vi "RF with WF Sweep.vi"() -> ()   [LabVIEW 2012]
uses:
  <vilib>/DAQmx/read.llb/DAQmx Read (Counter U32 1Chan 1Samp).vi
  <vilib>/Utility/file.llb/Write To Spreadsheet File (DBL).vi
  <vilib>/DAQmx/miscellaneous.llb/DAQmx Fill In Error Info.vi
  <vilib>/DAQmx/create/channels.llb/DAQmx Create Channel (CI-Count Edges).vi
  <vilib>/DAQmx/create/channels.llb/DAQmx Create Channel (CO-Pulse Generation-Ticks).vi
  <vilib>/DAQmx/configure/timing.llb/DAQmx Timing (Implicit).vi
  <vilib>/DAQmx/configure/timing.llb/DAQmx Timing (Sample Clock).vi
  <resource>/objmgr/daqmx.rc
panel:
  out "Scan":i32=222
  in  "N Scans":i32=100
  out "freq":dbl=349000000.0
  out "diff":dbl=487.0
  out "loop":i32=99
  in  "file path (dialog if empty)":path
  out "Z Position 2":dbl=39.24
  out "Y Position 2":dbl=141.00216667506004
  out "X Position 2":dbl=-28.668339852561274
  in  "CW for tracking":bool
  in  "Y Parameters":T1={"Number of Y Steps"=200, "Max Y (V)"=2.0, "Min Y (V)"=-2.0}
  in  "X":T2={"Number of X Steps"=200, "Max X (V)"=2.0, "Min X (V)"=-2.0}
  in  "Z Position":dbl=39.24
  in  "Y Position":dbl=136.0
  in  "X Position":dbl=-24.0
  in  "Z-track?":bool=TRUE
  out "XY Graph":cluster{"Y":dbl[], "Y":dbl[]}[](graph)=[{"Y"=[250000000.0, 251000000.0, 252000000.0, 253000000.0, 254000000.0, 255000000.0, 256000000.0, 257000000.0, 258000000.0, 259000000.0, 260000000.0, 261000000.0, 262000000.0, 263000000.0, 264000000.0, 265000000.0, 266000000.0, 267000000.0, 268000000.0, 269000000.0, 270000000.0, 271000000.0, 272000000.0, 273000000.0, 274000000.0, 275000000.0, 276000000.0, 277000000.0, 278000000.0, 279000000.0, 280000000.0, 281000000.0, 282000000.0, 283000000.0, 284000000.0, 285000000.0, 286000000.0, 287000000.0, 288000000.0, 289000000.0, 290000000.0, 291000000.0, 292000000.0, 293000000.0, 294000000.0, 295000000.0, 296000000.0, 297000000.0, 298000000.0, 299000000.0, 300000000.0, 301000000.0, 302000000.0, 303000000.0, 304000000.0, 305000000.0, 306000000.0, 307000000.0, 308000000.0, 309000000.0, 310000000.0, 311000000.0, 312000000.0, 313000000.0, 314000000.0, 315000000.0, 316000000.0, 317000000.0, 318000000.0, 319000000.0, 320000000.0, 321000000.0, 322000000.0, 323000000.0, 324000000.0, 325000000.0, 326000000.0, 327000000.0, 328000000.0, 329000000.0, 330000000.0, 331000000.0, 332000000.0, 333000000.0, 334000000.0, 335000000.0, 336000000.0, 337000000.0, 338000000.0, 339000000.0, 340000000.0, 341000000.0, 342000000.0, 343000000.0, 344000000.0, 345000000.0, 346000000.0, 347000000.0, 348000000.0, 349000000.0], "Y"=[109367.0, 118171.0, 118039.0, 118323.0, 118900.0, 117820.0, 117949.0, 118621.0, 118408.0, 118705.0, 117982.0, 118762.0, 119039.0, 119174.0, 119042.0, 119150.0, 118801.0, 118275.0, 118226.0, 119115.0, 118390.0, 118344.0, 118771.0, 118925.0, 118432.0, 118761.0, 118837.0, 118494.0, 117973.0, 117930.0, 118009.0, 118829.0, 118281.0, 119222.0, 118046.0, 117569.0, 117633.0, 117115.0, 116624.0, 116136.0, 115617.0, 116138.0, 116137.0, 116297.0, 115963.0, 116921.0, 117750.0, 117966.0, 118454.0, 117806.0, 117382.0, 116437.0, 117111.0, 116829.0, 116627.0, 115825.0, 116660.0, 116366.0, 116608.0, 116374.0, 116876.0, 116660.0, 117066.0, 116940.0, 116833.0, 117718.0, 117672.0, 118037.0, 118493.0, 118553.0, 118497.0, 117416.0, 118662.0, 117772.0, 118756.0, 117519.0, 117715.0, 118588.0, 117434.0, 117658.0, 117836.0, 118066.0, 118672.0, 118019.0, 118259.0, 118223.0, 118716.0, 118339.0, 117569.0, 118481.0, 118298.0, 118509.0, 118430.0, 117846.0, 117520.0, 117628.0, 118067.0, 118519.0, 118455.0, 117629.0]}]
  in  "Freq Max":dbl=350000000.0
  in  "Freq  Step":dbl=1000000.0
  in  "Freq Min":dbl=250000000.0
  in  "power":dbl=-9.0
  in  "stop":bool
  in  "Path to spinapi.dll":path=path "C:/SpinCore/SpinAPI/dll/spinapi64.dll"
  in  "Pulse offset":dbl
  in  "Tau":dbl=5e-07
  in  "RF Pulse":dbl=1e-07
  in  "Rabi Freq":dbl=11750000.0
  in  "MW Delay":dbl=2e-08
  in  "APD signal width":dbl=3e-07
  in  "Signal Delay":dbl=7.6e-07
  in  "AOM Rest time":dbl=1e-06
  in  "AOM Pulse length":dbl=2.5e-06
  in  "N Loop":i32=100000
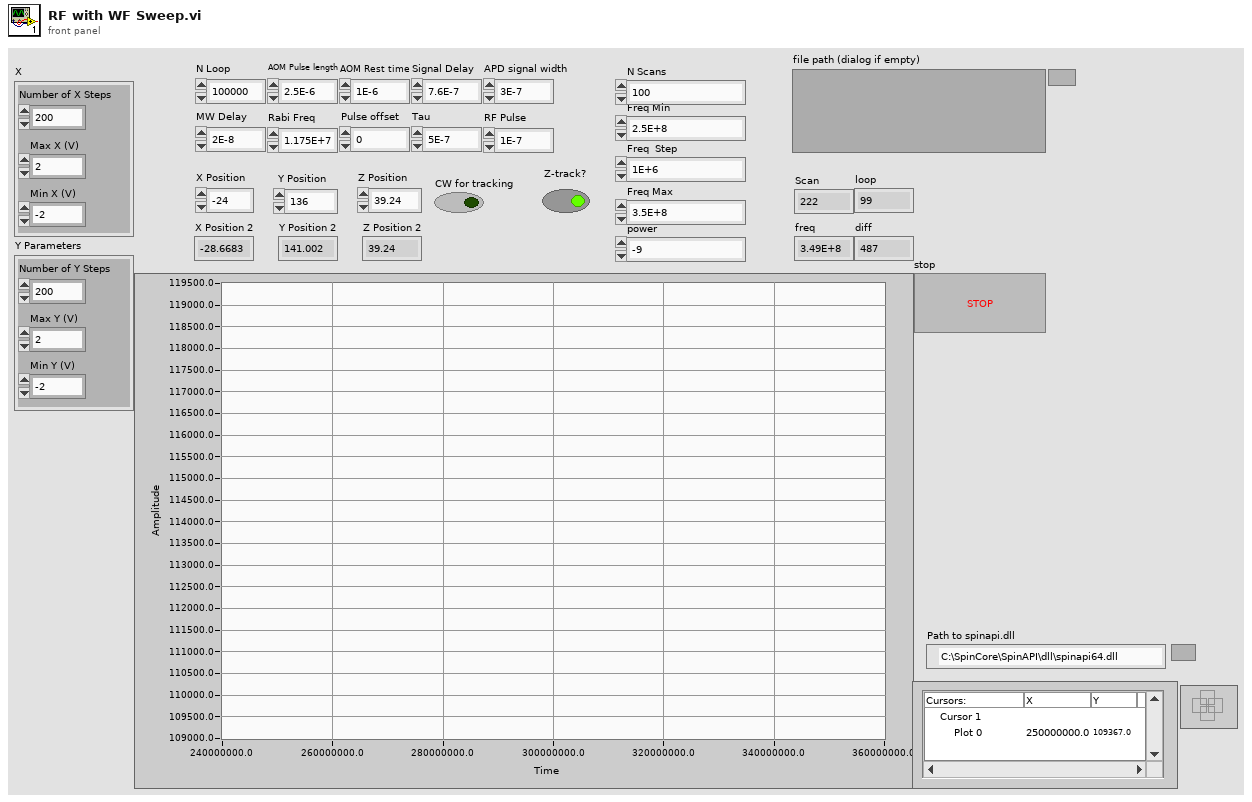
[diagram p1: front panel]
types:
  T1 = cluster{"Number of Y Steps":i32, "Max Y (V)":dbl, "Min Y (V)":dbl}
  T2 = cluster{"Number of X Steps":i32, "Max X (V)":dbl, "Min X (V)":dbl}
  T3 = enum16{"Pulse Program", "Frequency Registers", "TX Phase Registers", "RX Phase Registers"}
  T4 = cluster{"Instruct Data":i32, "Op Code":i32, "Flags":bool[], "Comments":string, "Time (s)":dbl}[]
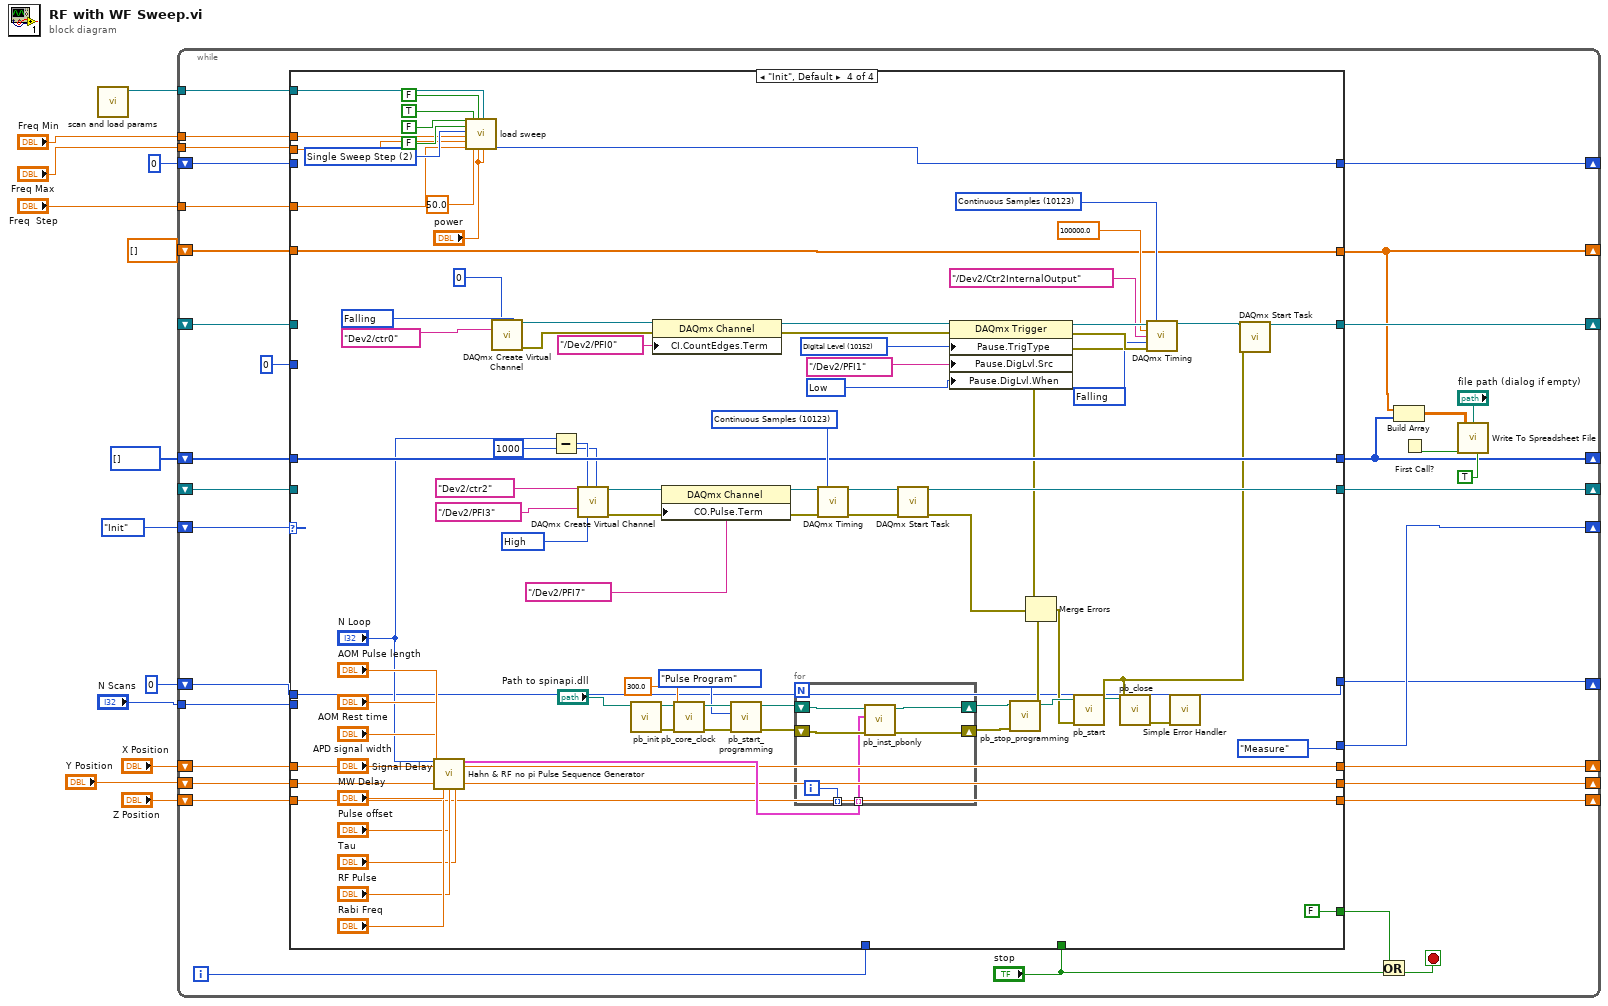
[diagram p0: block diagram]
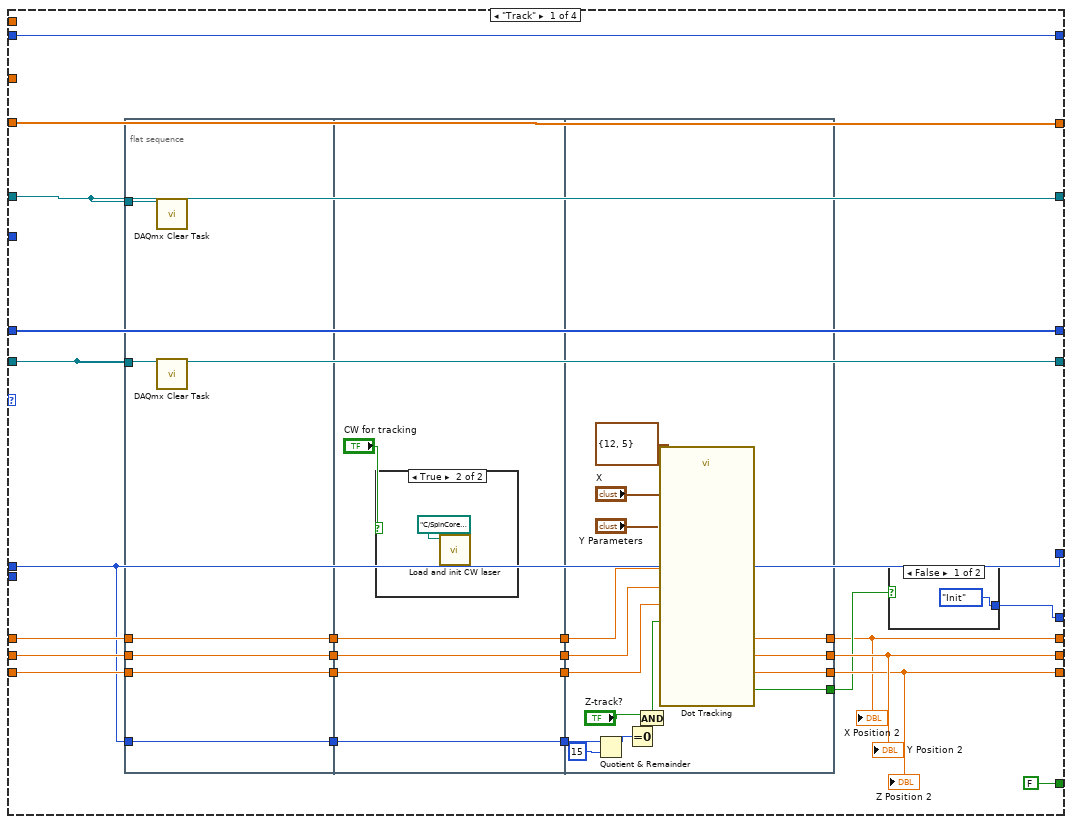
[diagram p2: hidden frame]
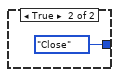
[diagram p3: hidden frame]
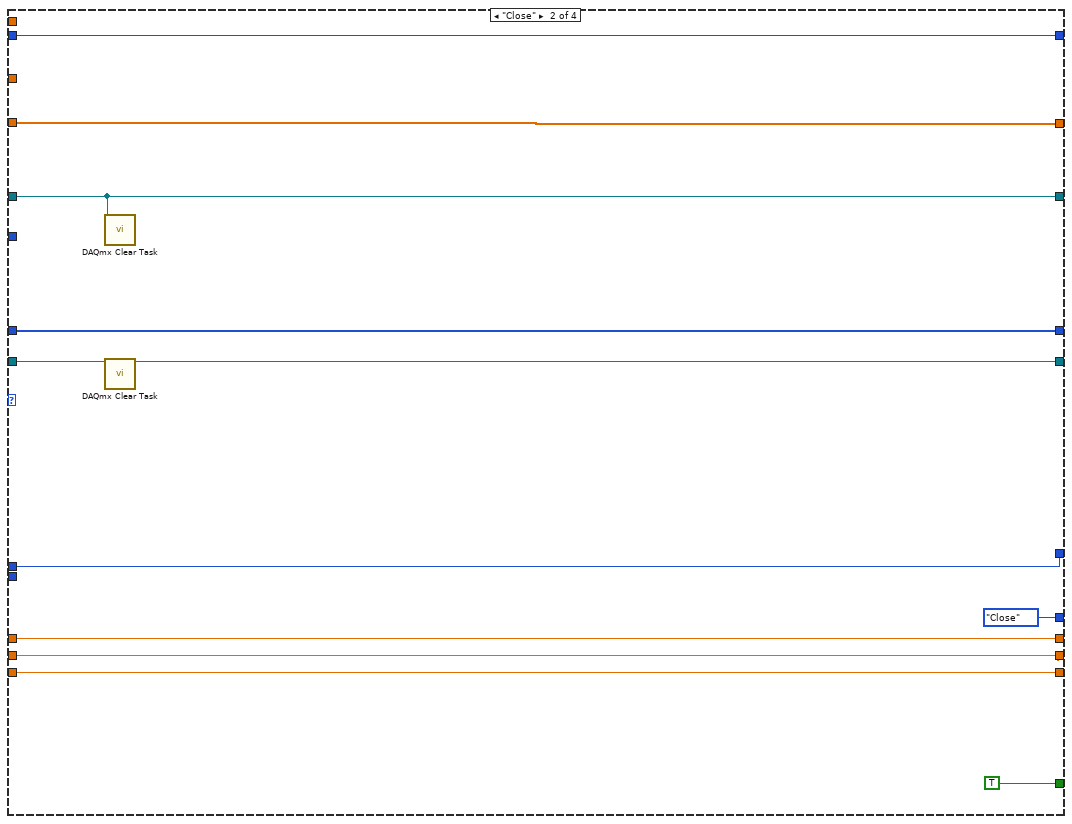
[diagram p5: hidden frame]
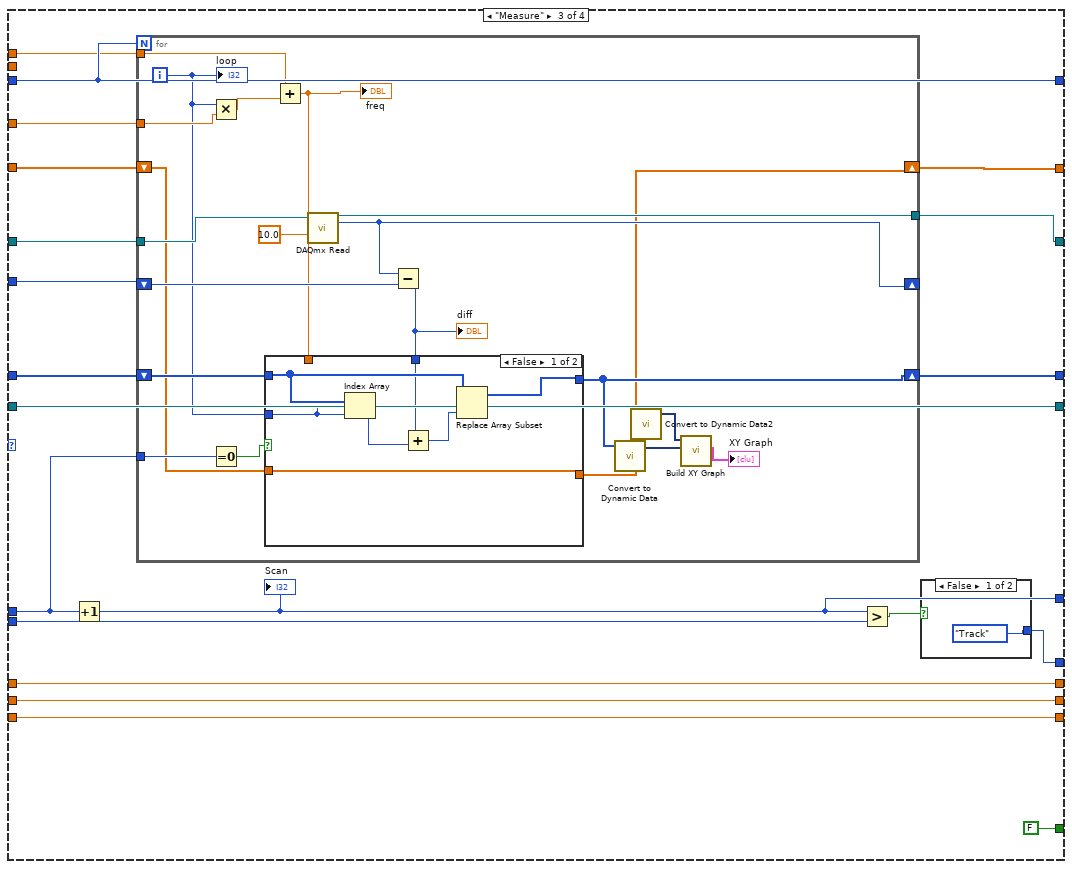
[diagram p6: hidden frame]
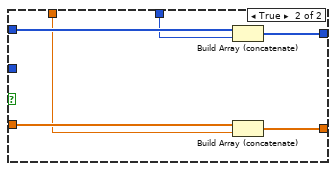
[diagram p7: hidden frame]
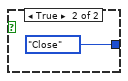
[diagram p8: hidden frame]
diagram:
  n1 = call "scan and load params.vi"() -> ("Serial Port Select"=w7:refnum<visa-resource-name>)  [unwired: 9 out]
  n2 = while {
    shift-right: [w41] -> _
    shift-left: enum16{"Init", "Track", "Measure", "Close", ""}."Init" -> [w47]
    shift-right: [w46] -> _
    shift-left: _ -> [w34]
    shift-right: [w45] -> _
    shift-left: _ -> [w35]
    shift-right: [w16] -> _
    shift-left: u32[] [] -> [w43]
    shift-right: [w29] -> _
    shift-left: dbl[] [] -> [w42]
    shift-right: [w40] -> _
    shift-left: "X Position" -> [w31]
    shift-right: [w39] -> _
    shift-left: "Y Position" -> [w37]
    shift-right: [w38] -> _
    shift-left: "Z Position" -> [w36]
    tunnel: w7 -> [w24]
    tunnel: "Freq  Step" -> [w21]
    tunnel: "Freq Max" -> [w22]
    tunnel: "Freq Min" -> [w23]
    shift-right: [w20] -> _
    shift-left: u16 0 ("Number\nof Points") -> [w19]
    tunnel: "N Scans" -> [w18]
    shift-right: [w15] -> _
    shift-left: 0 -> [w17]
    i -> [w14]
    stop <- w33 stop-if-true
    n3 = case shown="\"Init\", Default" w47 {
      tunnel: [w54 w111 w125 w196] -> w46
      tunnel: [w53 w110 w118 w195] -> w45
      tunnel: "stop" -> [_ _ _ _]
      tunnel: w43 -> [w63 w109 w131 w193]
      tunnel: w42 -> [w58 w104 w130 w189]
      tunnel: [w63 w109 w129 w193] -> w16
      tunnel: [w58 w104 w122 w189] -> w29
      tunnel: [w62 enum16{"Init", "Track", "Measure", "Close", ""}."Close" w128 enum16{"Init", "Track", "Measure", "Close", ""}."Measure"] -> w41
      tunnel: [w51 w103 w121 w188] -> w40
      tunnel: [w70 w108 w124 w191] -> w39
      tunnel: [w69 w107 w123 w190] -> w38
      tunnel: w37 -> [w66 w108 w124 w191]
      tunnel: w36 -> [w64 w107 w123 w190]
      tunnel: w35 -> [w53 w110 w126 _]
      tunnel: w34 -> [w54 w111 w125 _]
      tunnel: [FALSE TRUE FALSE FALSE] -> w32
      tunnel: w31 -> [w59 w103 w121 w188]
      tunnel: u32 0 ("data") -> [_ _ w120 _]
      tunnel: w24 -> [_ _ _ w181]
      tunnel: w23 -> [_ _ w117 w173]
      tunnel: w22 -> [_ _ _ w172]
      tunnel: w21 -> [_ _ w116 w171]
      tunnel: [w52 w102 w119 w170] -> w20
      tunnel: w19 -> [w52 w102 w119 _]
      tunnel: w18 -> [_ _ w114 _]
      tunnel: w17 -> [w50 w101 w112 w169]
      tunnel: [w50 w101 w113 w169] -> w15
      tunnel: w14 -> [_ _ _ _]
      frame "Track" {
        n4 = flat-sequence {
          tunnel: w64 -> [w76]
          tunnel: w66 -> [w77]
          tunnel: w59 -> [w78]
          tunnel: [w78] -> w57
          tunnel: [w77] -> w56
          tunnel: [w76] -> w55
          tunnel: w54 -> [w75]
          tunnel: w53 -> [w74]
          tunnel: w50 -> [w73]
          tunnel: [w73] -> w49
          tunnel: [w83] -> w68
          tunnel: [w82] -> w67
          tunnel: [w81] -> w65
          tunnel: w57 -> [w83]
          tunnel: w56 -> [w82]
          tunnel: w55 -> [w81]
          tunnel: w49 -> [w79]
          tunnel: [w79] -> w48
          tunnel: [w100] -> w51
          tunnel: [w99] -> w70
          tunnel: [w98] -> w69
          tunnel: w68 -> [w97]
          tunnel: w67 -> [w96]
          tunnel: w65 -> [w95]
          tunnel: [w91] -> w61
          tunnel: w48 -> [w85]
          frame #0 {
            n5 = call <vilib>:"DAQmx Clear Task.vi"("task in"=w74) -> ()  [unwired: 14 in, 1 out]
            n6 = call <vilib>:"DAQmx Clear Task.vi"("task in"=w75) -> ()  [unwired: 14 in, 1 out]
          }
          frame #1 {
            n7 = case shown="True" "CW for tracking" {
              frame False {
              }
              frame True {
                n8 = call "Load and init CW laser.vi"("path in"=path "C:/SpinCore/SpinAPI/dll/spinapi64.dll") -> ()  [unwired: 11 in]
              }
            }
          }
          frame #2 {
            n9 = Quotient & Remainder(x=w85, y=15) -> (x-y*floor(x/y)=w89:i32)  [unwired: 1 out]
            n10 = Equal To 0?(x=w89) -> (x = 0?=w88:bool)
            n11 = And(x="Z-track?", y=w88) -> (x .and. y?=w86:bool)
            n12 = call "Dot Tracking.vi"("X"="X", "Y Parameters"="Y Parameters", "RS232 settings"=cluster{"Portnumber":i32, "Baudrate":u16} {"Portnumber"=12, "Baudrate"=5}, "X Pos"=w97, "Y pos"=w96, "Z Pos"=w95, "Z-track?"=w86) -> ("X Position"=w100:dbl, "Y Position"=w99:dbl, "Z Position"=w98:dbl, "Gave up?"=w91:bool)  [unwired: 2 in, 3 out]
          }
        }
        n13 = case shown="False" w61 {
          tunnel: [enum16{"Init", "Track", "Measure", "Close", ""}."Init" enum16{"Init", "Track", "Measure", "Close", ""}."Close"] -> w62
          frame False {
          }
          frame True {
          }
        }
        "X Position 2" <- w51
        "Y Position 2" <- w70
        "Z Position 2" <- w69
      }
      frame "Close" {
        n14 = call <vilib>:"DAQmx Clear Task.vi"("task in"=w110) -> ()  [unwired: 14 in, 1 out]
        n15 = call <vilib>:"DAQmx Clear Task.vi"("task in"=w111) -> ()  [unwired: 14 in, 1 out]
      }
      frame "Measure" {
        n16 = Increment(x=w112) -> (x+1=w113:i32)
        "Scan" <- w113
        n17 = for {
          N: w119 -> [_]
          shift-right: [w142] -> w129
          shift-left: w131 -> [w143]
          shift-right: [w133] -> w122
          shift-left: w130 -> [w134]
          tunnel: w126 -> [w150]
          shift-right: [w145] -> _
          shift-left: w120 -> [w147]
          tunnel: [w146] -> w118
          tunnel: w117 -> [w141]
          tunnel: w116 -> [w140]
          tunnel: w112 -> [w137]
          i -> [w135]
          n18 = Multiply(x=w135, y=w140) -> (x*y=w139:dbl)
          n19 = Equal To 0?(x=w137) -> (x = 0?=w136:bool)
          n20 = Add(x=w141, y=w139) -> (x+y=w132:dbl)
          "freq" <- w132
          n21 = call-poly <vilib>:"DAQmx Read.vi"("task/channels in"=w150, "timeout"=10.0) -> ("task out"=w146:refnum<k21>, "data"=w145:u32)  [unwired: 11 in, 1 out]
          n22 = Subtract(x=w145, y=w147) -> (x-y=w138:u32)
          "diff" <- w138
          n23 = case shown="False" w136 {
            tunnel: w143 -> [w158 w164]
            tunnel: [w153 w163] -> w142
            tunnel: w138 -> [w155 w162]
            tunnel: w135 -> [w157 _]
            tunnel: w134 -> [w152 w161]
            tunnel: [w152 w160] -> w133
            tunnel: w132 -> [_ w159]
            frame False {
              n24 = Index Array(array=w158, index=w157) -> (element=w156:u32)
              n25 = Add(x=w155, y=w156) -> (x+y=w154:u32)
              n26 = Replace Array Subset(array=w158, new element=w154, index=w157) -> (w153:u32[])
            }
            frame True {
              n27 = Build Array (concatenate)(w164, w162) -> (w163:u32[])
              n28 = Build Array (concatenate)(w161, w159) -> (w160:dbl[])
            }
          }
          n29 = call "Convert to Dynamic Data"("Array"=w142) -> ("Dynamic Data Type"=w148:dynamicdata)  [unwired: 3 in]
          n30 = call "Convert to Dynamic Data2"("Array"=w133) -> ("Dynamic Data Type"=w149:dynamicdata)  [unwired: 3 in]
          n31 = call "Build XY Graph"("Y Input"=w148, "X Input"=w149) -> ("XY Graph"=→"XY Graph":cluster{"Y":dbl[], "Y":dbl[]}[])  [unwired: 3 in, 6 out]
          "loop" <- w135
        }
        n32 = Greater?(x=w113, y=w114) -> (0:w115:bool)
        n33 = case shown="False" w115 {
          tunnel: [enum16{"Init", "Track", "Measure", "Close", ""}."Track" enum16{"Init", "Track", "Measure", "Close", ""}."Close"] -> w128
          frame False {
          }
          frame True {
          }
        }
      }
      frame "Init", Default {
        w167 = 10171 items=["Rising"=10280, "Falling"=10171] ("active edge")
        w168 = 10192 items=["High"=10192, "Low"=10214] ("idle state")
        w176 = 2 items=["No Triggers", "Full Frequency Sweep", "Single Sweep Step", "Stop All", "Digital RF On/Off", "Remove Interrupts", "Reserved 1", "Reserved 2", "Ext AM Modulation", "Ext FM Modulation"] ("Trigger")
        w182 = 1000 ("y")
        w204 = 10123 items=["Finite Samples"=10178, "Continuous Samples"=10123, "Hardware Timed Single Point"=12522] ("sample mode")
        w222 = 10214 items=["High"=10192, "Low"=10214] ("Pause.DigLvl.When")
        w224 = 10152 items=["Analog Level"=10101, "Analog Window"=10103, "Digital Level"=10152, "Digital Pattern"=10398, "None"=10230] ("Pause.TrigType")
        w211 = 10123 items=["Finite Samples"=10178, "Continuous Samples"=10123, "Hardware Timed Single Point"=12522] ("sample mode")
        w200 = 10171 items=["Rising"=10280, "Falling"=10171] ("edge")
        n34 = call "Hahn & RF no pi Pulse Sequence Generator.vi"("N Loop"="N Loop", "Rabi Frequency"="Rabi Freq", "RF Pulse"="RF Pulse", "Tau"="Tau", "AOM Pulse length"="AOM Pulse length", "AOM Rest time"="AOM Rest time", "Signal Delay"="Signal Delay", "APD signal width"="APD signal width", "MW Delay"="MW Delay", "Pulse offset"="Pulse offset") -> ("Pulse Sequence"=w225:T4)  [unwired: 5 in]
        n35 = call "load sweep.vi"("Channel"=FALSE, "Sweep\nContinuously"=FALSE ("Sweep\nContinuously"), "Trigger"=w176, "Start Frequency"=w173, "Stop Frequency"=w172, "Step Size MHz"=w171, "RF On"=TRUE, "Step Time (mS)"=50.0, "load?"=FALSE, "Start Amplitude"="power", "Serial Port Select"=w181, "Stop Amplitude"="power") -> ("Number\nof Points"=w170:u16)  [unwired: 7 in]
        n36 = call-poly <vilib>:"DAQmx Create Virtual Channel.vi"("initial count"=u32 0, "edge"=w200, "counter"=tag "Dev2/ctr0") -> ("task out"=w220:refnum<k21>, "error out"=w217:errorcluster)  [unwired: 6 in, 5 out]
        n37 = Subtract(x="N Loop", y=w182) -> (x-y=w184:i32)
        n38 = call-poly <vilib>:"DAQmx Create Virtual Channel.vi"("high ticks"=w184, "low ticks"=w182, "counter"=tag "Dev2/ctr2", "source of ticks"=tag "/Dev2/PFI3" ("source"), "idle state"=w168) -> ("task out"=w208:refnum<k21>, "error out"=w206:errorcluster)  [unwired: 9 in]
        n39 = call "pb_init.vi"("path in"="Path to spinapi.dll") -> ("error out"=w231:errorcluster, "path out"=w229:path)  [unwired: 3 in, 6 out]
        n40 = property class="DAQmx Channel"(reference=w220, error in=w217, "CI.CountEdges.Term"=tag "/Dev2/PFI0") -> (reference out=w221:refnum<k21>, error out=w219:errorcluster)
        n41 = property class="DAQmx Channel"(reference=w208, "CO.Pulse.Term"=tag "/Dev2/PFI7") -> (reference out=w203:refnum<k21>)  [unwired: 1 in, 1 out]
        n42 = call "pb_core_clock.vi"("error in (no error)"=w231, "clock_freq (MHz)"=300.0, "path in"=w229) -> ("error out"=w232:errorcluster, "path out"=w230:path)  [unwired: 7 in]
        n43 = call "pb_start_programming.vi"("error in (no error)"=w232, "Device"=T3."Pulse Program", "path in"=w230) -> ("error out"=w235:errorcluster, "path out"=w234:path)  [unwired: 1 in, 6 out]
        n44 = for {
          shift-right: [w252] -> w236
          shift-left: w234 -> [w254]
          shift-right: [w251] -> w237
          shift-left: w235 -> [w253]
          tunnel: [w250] -> _ mode=indexing
          tunnel: w225 -> [w249] mode=indexing
          i -> [w250]
          n45 = call "pb_inst_pbonly.vi"("error in (no error)"=w253, "PB Instruction"=w249, "path in"=w254) -> ("error out"=w251:errorcluster, "path out"=w252:path)  [unwired: 2 in, 5 out]
        }
        n46 = call-poly <vilib>:"DAQmx Timing.vi"("task/channels in"=w203, "sample mode"=w204, "error in"=w206) -> ("task out"=w207:refnum<k21>, "error out"=w205:errorcluster)  [unwired: 11 in]
        n47 = call <vilib>:"DAQmx Start Task.vi"("task/channels in"=w207, "error in"=w205) -> ("task out"=w196:refnum<k21>, "error out"=w199:errorcluster)  [unwired: 12 in]
        n48 = property class="DAQmx Trigger"(reference=w221, error in=w219, "Pause.TrigType"=w224, "Pause.DigLvl.Src"=tag "/Dev2/PFI1", "Pause.DigLvl.When"=w222) -> (reference out=w216:refnum<k21>, error out=w215:errorcluster)
        n49 = call "pb_stop_programming.vi"("error in (no error)"=w237, "path in"=w236) -> ("error out"=w197:errorcluster, "path out"=w227:path)  [unwired: 1 in, 7 out]
        n50 = call-poly <vilib>:"DAQmx Timing.vi"("task/channels in"=w216, "sample mode"=w211, "rate"=100000.0, "source"=tag "/Dev2/Ctr2InternalOutput", "active edge"=w167, "error in"=w215) -> ("task out"=w213:refnum<k21>, "error out"=w186:errorcluster)  [unwired: 8 in]
        n51 = Merge Errors(w186, w199, w197) -> (w198:errorcluster)
        n52 = call "pb_start.vi"("error in (no error)"=w198, "path in"=w227) -> ("error out"=w185:errorcluster, "path out"=w226:path)  [unwired: 1 in, 7 out]
        n53 = call "pb_close.vi"("error in (no error)"=w185, "path in"=w226) -> ("error out"=w239:errorcluster)  [unwired: 9 out]
        n54 = call <vilib>:"Simple Error Handler.vi"("error in (no error)"=w239) -> ()  [unwired: 1 in, 8 out]
        n55 = call <vilib>:"DAQmx Start Task.vi"("task/channels in"=w213, "error in"=w185) -> ("task out"=w195:refnum<k21>)  [unwired: 13 out]
      }
    }
    n56 = Or(x=w32, y="stop") -> (x .or. y?=w33:bool)
    n57 = Build Array(w29, w16) -> (w28:dbl[][])
    n58 = First Call?() -> (First Call?: T/F=w25:bool)
    n59 = call-poly <vilib>:"Write To Spreadsheet File.vi"("transpose? (no:F)"=TRUE, "append to file? (new file:F)"=w25, "2D data"=w28, "file path (dialog if empty)"="file path (dialog if empty)") -> ()  [unwired: 4 in, 1 out]
  }
